vi "Get URL Contents.vi"(8 "error in (no error)":errorcluster, 10 "TCP Timeout (3000 ms)":i32=3000, 11 "URL":string="http://macdailynews.com/index.php/weblog/rss_2.0") -> (0 "error out":errorcluster, 3 "Contents":string)   [LabVIEW 2020, in "Feed.lvclass"]
uses:
  <vilib>/NI_RSS/Feed/Feed.lvclass
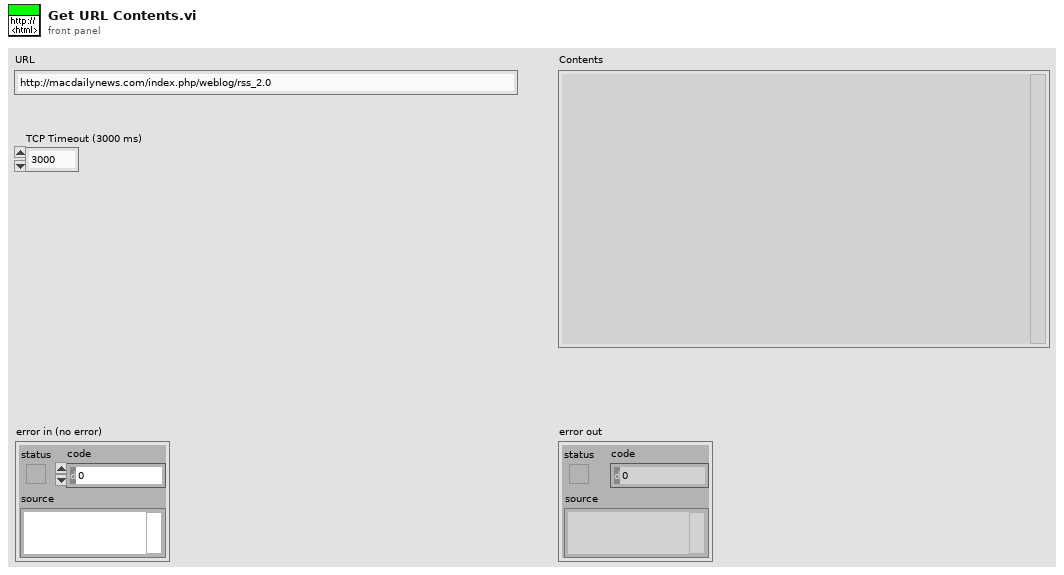
[diagram p1: front panel]
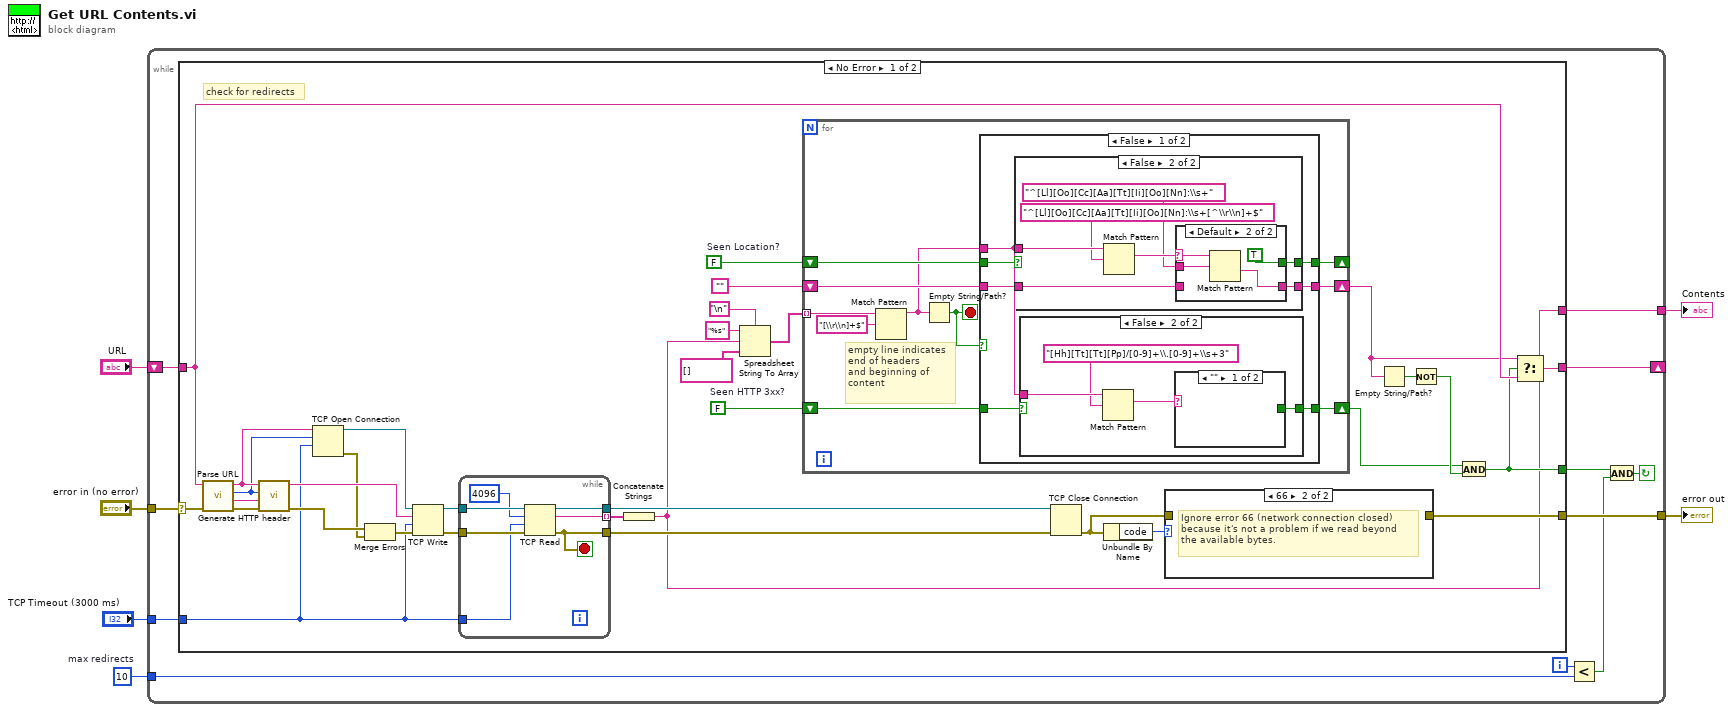
[diagram p0: block diagram]
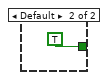
[diagram p3: hidden frame]
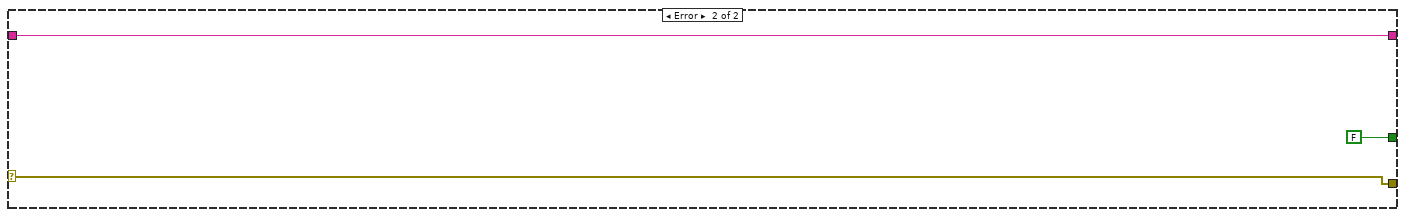
[diagram p8: hidden frame]
diagram:
  w2 = 10  # max redirects
  n1 = while {
    tunnel: [w16] -> w5
    tunnel: "error in (no error)" -> [w15]
    shift-right: [w13] -> _
    shift-left: "URL" -> [w17]
    tunnel: [w14] -> w3
    tunnel: w2 -> [w10]
    tunnel: "TCP Timeout (3000 ms)" -> [w7]
    i -> [w11]
    stop <- w8 continue-if-true
    n2 = case shown="No Error" w15 {
      selector: w15 -> [w35 w102]
      tunnel: w17 -> [w32 w101]
      tunnel: [w22 _] -> w14
      tunnel: [w36 w102] -> w16
      tunnel: [w31 w101] -> w13
      tunnel: [w30 FALSE] -> w12
      tunnel: w7 -> [w18 _]
      frame No Error {
        w26 = FALSE  # Seen HTTP 3xx?
        w29 = FALSE  # Seen Location?
        # "check for redirects"
        n3 = call <vilib>:"Parse URL.vi"("error in (no error)"=w35, "URL"=w32) -> ("error out"=w50:errorcluster, "Path"=w51:string, "Port"=w48:i32, "Server"=w49:string)  [unwired: 6 out]
        n4 = call <vilib>:"Generate HTTP header.vi"("error out"=w50, "Path"=w51, "Port"=w48, "Server"=w49) -> ("error IO"=w45:errorcluster, "HTTP Header"=w46:string)  [unwired: 2 out]
        n5 = TCP Open Connection(address=w49, remote port or service name=w48, timeout ms (60000)=w18) -> (connection ID=w47:refnum<k5>, error out=w44:errorcluster)  [unwired: 1 in, 1 out]
        n6 = Merge Errors(w45, w44) -> (w43:errorcluster)
        n7 = TCP Write(connection ID=w47, data in=w46, error in (no error)=w43, 9:w18) -> (connection ID out=w42:refnum<k5>, error out=w41:errorcluster)  [unwired: 1 out]
        n8 = while {
          tunnel: w42 -> [w58]
          tunnel: w41 -> [w57]
          tunnel: [w54] -> w23 mode=indexing
          tunnel: [w56] -> w38
          tunnel: [w55] -> w40
          tunnel: w18 -> [w52]
          stop <- w56 stop-if-true
          n9 = TCP Read(connection ID=w58, bytes to read=4096, error in (no error)=w57, 9:w52) -> (connection ID out=w55:refnum<k5>, data out=w54:string, error out=w56:errorcluster)  [unwired: 1 out]
        }
        n10 = Concatenate Strings(w23) -> (w22:string)
        n11 = Spreadsheet String To Array(delimiter (Tab)="\n", format string="%s", spreadsheet string=w22, array type (2D Dbl)=string[] []) -> (array=w24:string[])
        n12 = for {
          tunnel: w24 -> [w62] mode=indexing
          shift-right: [w65] -> _
          shift-left: w29 -> [w68]
          shift-right: [w66] -> w27
          shift-left: "" -> [w67]
          shift-right: [w63] -> w25
          shift-left: w26 -> [w64]
          stop <- w59 stop-if-true
          # "empty line indicates\nend of headers\nand beginning of\ncontent"
          n13 = Match Pattern(string=w62, regular expression="[\\r\\n]+$") -> (before substring=w60:string)  [unwired: 1 in, 3 out]
          n14 = Empty String/Path?(string/path=w60) -> (empty?=w59:bool)
          n15 = case shown="False" w59 {
            tunnel: w68 -> [w75 w97]
            tunnel: w67 -> [w74 w98]
            tunnel: [w73 w98] -> w66
            tunnel: [w72 w97] -> w65
            tunnel: w60 -> [w71 _]
            tunnel: w64 -> [w70 w96]
            tunnel: [w69 w96] -> w63
            frame False {
              n16 = case shown="False" w75 {
                selector: w75 -> [w83 _]
                tunnel: w71 -> [_ w90]
                tunnel: w74 -> [w82 w86]
                tunnel: [w82 w85] -> w73
                tunnel: [w83 w84] -> w72
                frame True {
                }
                frame False {
                  n17 = Match Pattern(string=w90, regular expression="^[Ll][Oo][Cc][Aa][Tt][Ii][Oo][Nn]:\\s+[^\\r\\n]+$") -> (match substring=w88:string)  [unwired: 1 in, 3 out]
                  n18 = case shown="Default" w88 {
                    selector: w88 -> [_ w95]
                    tunnel: [w91 w94] -> w85
                    tunnel: "^[Ll][Oo][Cc][Aa][Tt][Ii][Oo][Nn]:\\s+" ("regular expression") -> [_ w93]
                    tunnel: w86 -> [w91 _]
                    tunnel: [_ TRUE] -> w84
                    frame "" {
                    }
                    frame Default {
                      n19 = Match Pattern(string=w95, regular expression=w93) -> (after substring=w94:string)  [unwired: 1 in, 3 out]
                    }
                  }
                }
              }
              n20 = case shown="False" w70 {
                selector: w70 -> [w76 _]
                tunnel: w71 -> [_ w80]
                tunnel: [w76 w77] -> w69
                frame True {
                }
                frame False {
                  n21 = Match Pattern(string=w80, regular expression="[Hh][Tt][Tt][Pp]/[0-9]+\\.[0-9]+\\s+3") -> (match substring=w78:string)  [unwired: 1 in, 3 out]
                  n22 = case shown="\"\"" w78 {
                    tunnel: [_ TRUE] -> w77
                    frame "" {
                    }
                    frame Default {
                    }
                  }
                }
              }
            }
            frame True {
            }
          }
        }
        n23 = TCP Close Connection(connection ID=w40, error in (no error)=w38) -> (error out=w37:errorcluster)  [unwired: 2 out]
        n24 = Unbundle By Name(w37) -> ("code"=w39:i32)
        n25 = case shown="66" w39 {
          tunnel: w37 -> [w99 _]
          tunnel: [w99 _] -> w36
          frame Default {
          }
          frame 66 {
            # "Ignore error 66 (network connection closed)\nbecause it's not a problem if we read beyond\nthe available bytes."
          }
        }
        n26 = Empty String/Path?(string/path=w27) -> (empty?=w34:bool)
        n27 = Not(x=w34) -> (.not. x?=w33:bool)
        n28 = And(x=w25, y=w33) -> (x .and. y?=w30:bool)
        n29 = Select(t=w27, s=w30, f=w32) -> (s? t:f=w31:string)
      }
      frame Error {
      }
    }
    n30 = Less?(x=w11, y=w10) -> (x < y?=w9:bool)
    n31 = And(x=w12, y=w9) -> (x .and. y?=w8:bool)
  }
  "Contents" <- w3
  "error out" <- w5
